vi "WRP Get Property String.vi"(8 "error in (no error)":errorcluster, 9 "size":i32, 10 "index":i32, 11 "property":string) -> (0 "error out":errorcluster, 1 "size out":i32, 2 "function return":i32, 3 "value":string)   [LabVIEW 2018, in "SesWrapper.lvlib"]
doc: "int STDCALL WRP_GetPropertyString(const String property, int index, String value, int *size);"
uses:
  SesWrapper.lvlib
  build/Debug/SESWrapper.dll
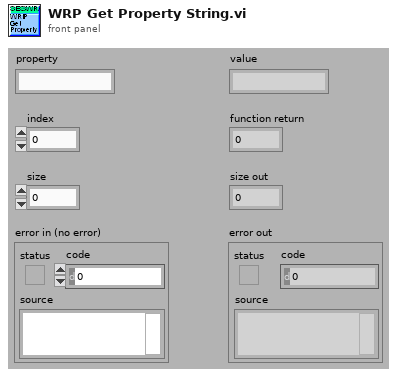
[diagram p1: front panel]
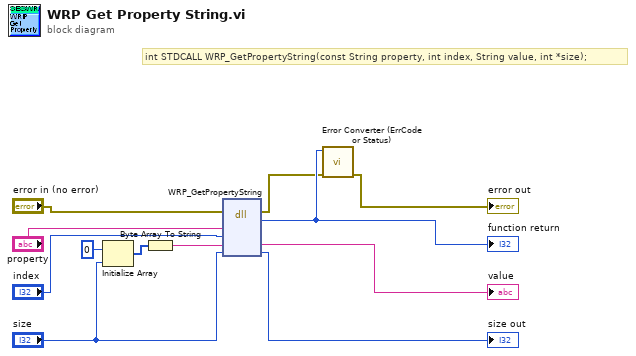
[diagram p0: block diagram]
diagram:
  # "int STDCALL WRP_GetPropertyString(const String property, int index, String value, int *size);"
  n1 = Initialize Array(u8 0 ("element"), "size") -> (w9:u8[])
  n2 = Byte Array To String(unsigned byte array=w9) -> (string=w8:string)
  n3 = dll-call lib="C:/Development/svn/seswrapper-lib/build/Debug/SESWrapper.*" fn="WRP_GetPropertyString"(error in="error in (no error)", "property"="property", "index"="index", "value"=w8, "size"="size") -> (error out=w2:errorcluster, w12:i32, "value"=→"value":string, "size"=→"size out":i32)  [unwired: 4 in, 1 out]
  "function return" <- w12
  n4 = call "Error Converter (ErrCode or Status).vi"("error in (no error)"=w2, "error code"=w12) -> ("error out"=→"error out":errorcluster)  [unwired: 9 in]
